vi "OnDrop.vi"(0 "XRef":T10, 1 "State In":T1 {"BlockNodeState"."Draw Style" items=["FunctionBlock", "ExpressVI", "Variable", "Elemental I/O", "32x32 Icon", "FunctionBlockCompact"]; "BlockNodeState"."Terminal Data"."Terminal Flags" format="%.0b"}) -> (14 "Reply":T8, 15 "State Out":T1 {"BlockNodeState"."Draw Style" items=["FunctionBlock", "ExpressVI", "Variable", "Elemental I/O", "32x32 Icon", "FunctionBlockCompact"]; "BlockNodeState"."Terminal Data"."Terminal Flags" format="%.0b"})   [LabVIEW 2020, in "Set DDT Attributes.lvlib" / "Set DDT Properties.xnode"]
uses:
  <vilib>/express/express signal manip/GetorSetDDTAttributes/Set DDT Attributes/Set DDT Properties.xnode
  <vilib>/XNodeSupport/XNodeXNodeRef.ctl
  <vilib>/express/express signal manip/GetorSetDDTAttributes/Set DDT Attributes/State.ctl
  <vilib>/BlockNodeSupport/BlockNodeState.ctl
  <vilib>/BlockNodeSupport/TerminalData.ctl
  <vilib>/picture/picture.llb/imagedata.ctl
  <vilib>/express/express signal manip/GetorSetDDTAttributes/Shared VIs/Attributes data.ctl
  <vilib>/express/express signal manip/GetorSetDDTAttributes/Shared VIs/Input.ctl
  <vilib>/express/express signal manip/GetorSetDDTAttributes/Shared VIs/Attributes name.ctl
  <vilib>/XNodeSupport/XNodeStringArray.ctl
  <vilib>/XNodeSupport/XNodeString.ctl
  <vilib>/XNodeSupport/NI_XNodeSupport.lvlib
  <vilib>/express/express signal manip/GetorSetDDTAttributes/Set DDT Attributes/Set DDT Attributes.lvlib
  <vilib>/express/express signal manip/GetorSetDDTAttributes/Shared VIs/GetSetShared.lvlib
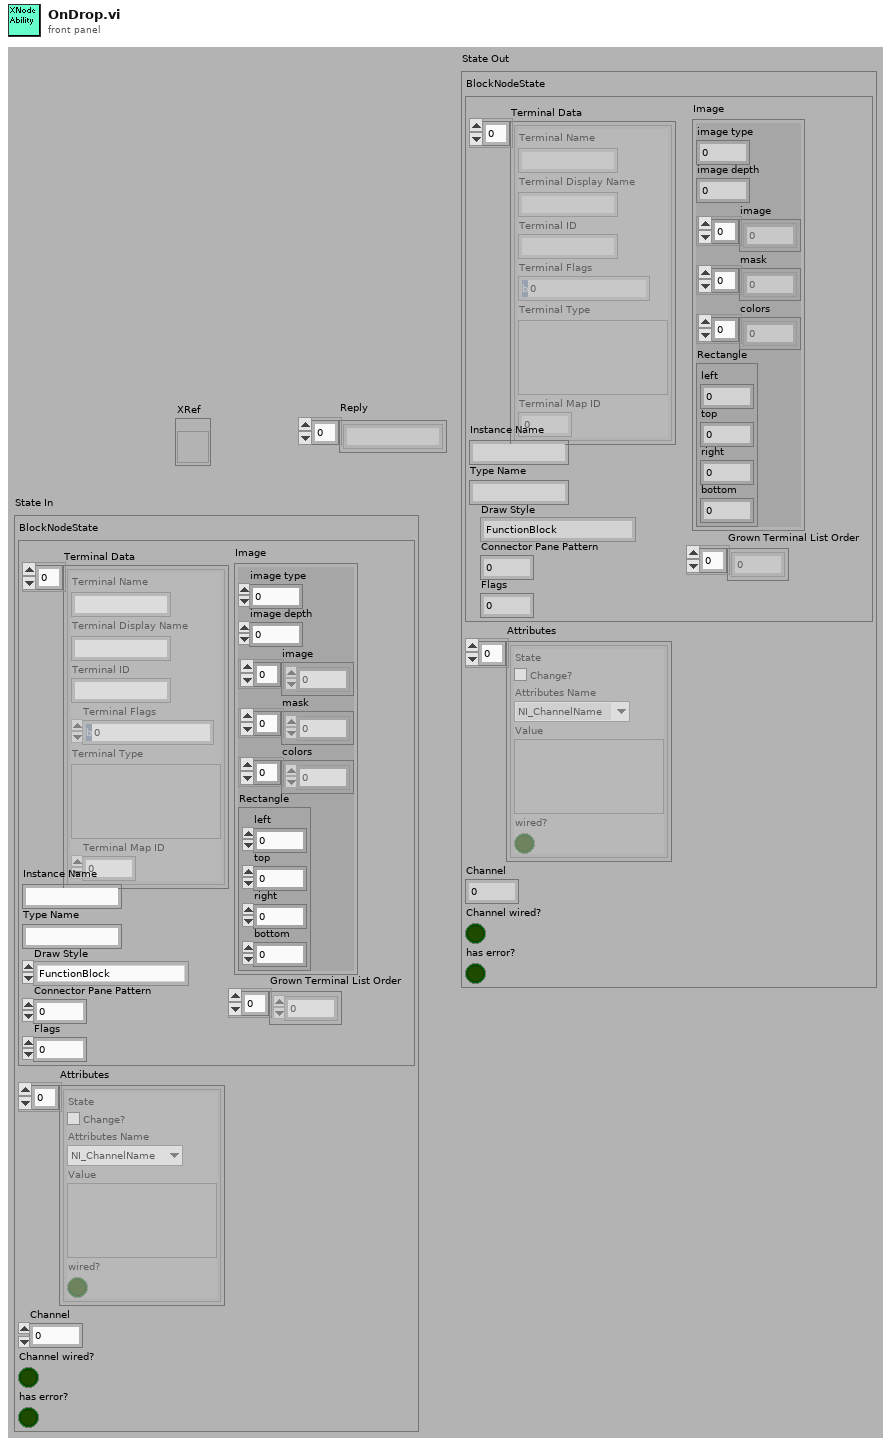
[diagram p1: front panel]
types:
  T1 = typedef "Set DDT Attributes.lvlib/Set DDT Properties.xnode/State.ctl" = cluster{"BlockNodeState":T2, "Attributes":T5[], "Channel":u32, "Channel wired?":bool, "has error?":bool}
  T2 = typedef "BlockNodeState.ctl" = cluster{"Terminal Data":T3[], "Instance Name":string, "Type Name":string, "Draw Style":i32, "Connector Pane Pattern":i32, "Flags":i32, "Grown Terminal List Order":i32[], "Image":T4}
  T3 = typedef "TerminalData.ctl" = cluster{"Terminal Name":string, "Terminal Display Name":string, "Terminal ID":string, "Terminal Flags":i32, "Terminal Type":variant, "Terminal Map ID":i32}
  T4 = typedef "imagedata.ctl" = cluster{"image type":i32, "image depth":i32, "image":u8[], "mask":u8[], "colors":u32[], "Rectangle":cluster{"left":i16, "top":i16, "right":i16, "bottom":i16}}
  T5 = typedef "GetSetShared.lvlib/Attributes data.ctl" = cluster{"State":T6, "Attributes Name":T7, "Value":variant, "wired?":bool}
  T6 = typedef "GetSetShared.lvlib/Input.ctl" = bool
  T7 = typedef "GetSetShared.lvlib/Attributes name.ctl" = enum16{"NI_ChannelName", "NI_ExpIsRelativeTime", "NI_ExpTimeStamp", "NI_ExpStartTimeStamp", "NI_ExpXDimension", "NI_UnitDescription"}
  T8 = typedef "NI_XNodeSupport.lvlib/XNodeStringArray.ctl" = T9[]
  T9 = typedef "NI_XNodeSupport.lvlib/XNodeString.ctl" = string
  T10 = typedef "NI_XNodeSupport.lvlib/XNodeXNodeRef.ctl" = refnum<vi>
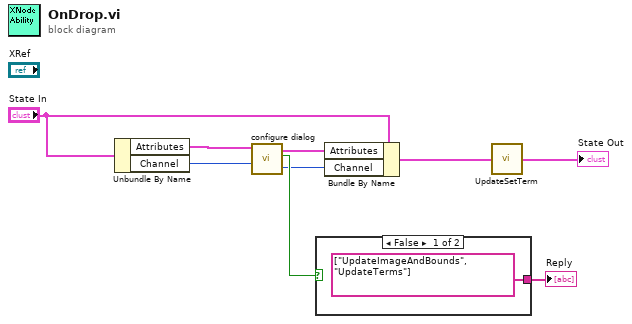
[diagram p0: block diagram]
diagram:
  n1 = Unbundle By Name("State In") -> ("Attributes"=w8:T5[], "Channel"=w5:u32)
  n2 = call <vilib>:"configure dialog.vi"("Channel"=w5, "Attributes in"=w8) -> ("Channel out"=w3:u32, "Cancelled?"=w4:bool, "Attributes out"=w7:T5[])  [unwired: 2 in, 5 out]
  n3 = case shown="False" w4 {
    tunnel: [T8 ["UpdateImageAndBounds", "UpdateTerms"] ("Reply") _] -> w9
    frame False {
    }
    frame True {
    }
  }
  "Reply" <- w9
  n4 = Bundle By Name(cluster="State In", "Attributes"=w7, "Channel"=w3) -> (w1:T1)
  n5 = call <vilib>:"UpdateSetTerm.vi"("State In"=w1) -> ("State Out"=→"State Out":T1)  [unwired: 1 in, 1 out]
